vi "HW_GEN - Read DevicesInfo from XML File.vi"(8 "error in":errorcluster caption="错误输入（无错误）", 11 "path to XML document":path=path "E:/00. 系统集成/000000 SignalPro/SourceCodes/Builds/Files/HWdef.xml" caption="XML文档路径") -> (0 "error out":errorcluster caption="错误输出", 2 "DevInfo[]":T1[](array[typedef]))   [LabVIEW 2016]
uses:
  <vilib>/xml/NI_XML.lvlib
  Ctrls/HardWare Basic Info _ Channel.ctl
  Ctrls/HardWare Basic Info _ Module.ctl
  Ctrls/HardWare Basic Info _ Chassis.ctl
  Ctrls/HardWare Basic Info _ Device.ctl
  <vilib>/xml/Load XML File.vi
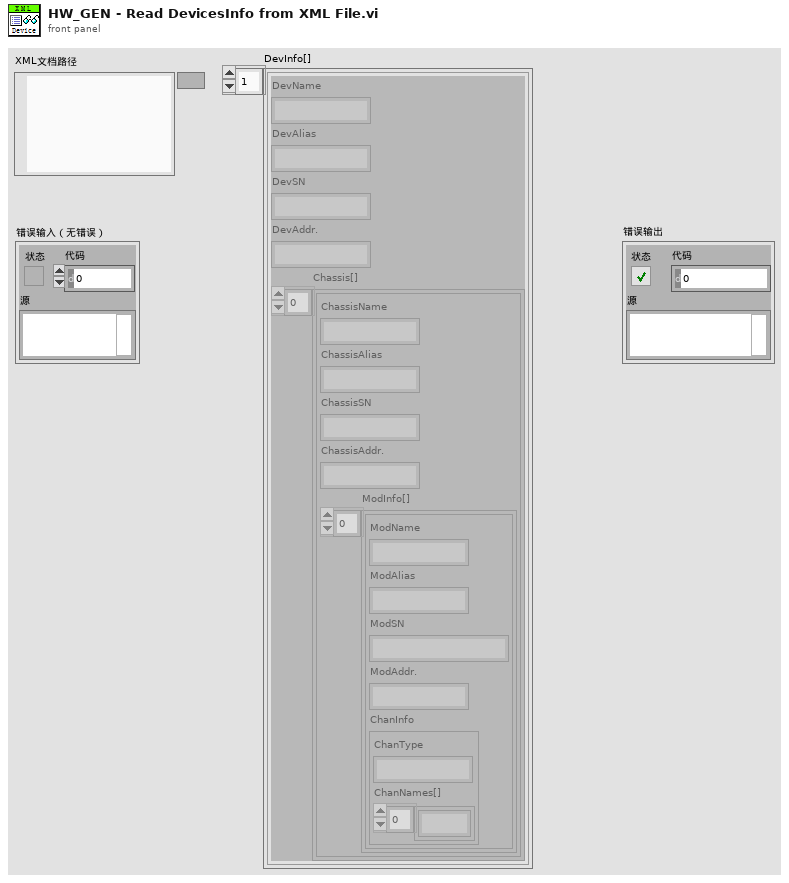
[diagram p1: front panel]
types:
  T1 = typedef "HardWare Basic Info _ Device.ctl" = cluster{"DevName":string, "DevAlias":string, "DevSN":string, "DevAddr.":string, "Chassis[]":T2[]}
  T2 = typedef "HardWare Basic Info _ Chassis.ctl" = cluster{"ChassisName":string, "ChassisAlias":string, "ChassisSN":string, "ChassisAddr.":string, "ModInfo[]":T3[]}
  T3 = typedef "HardWare Basic Info _ Module.ctl" = cluster{"ModName":string, "ModAlias":string, "ModSN":string, "ModAddr.":string, "ChanInfo":T4}
  T4 = typedef "HardWare Basic Info _ Channel.ctl" = cluster{"ChanType":string, "ChanNames[]":string[]}
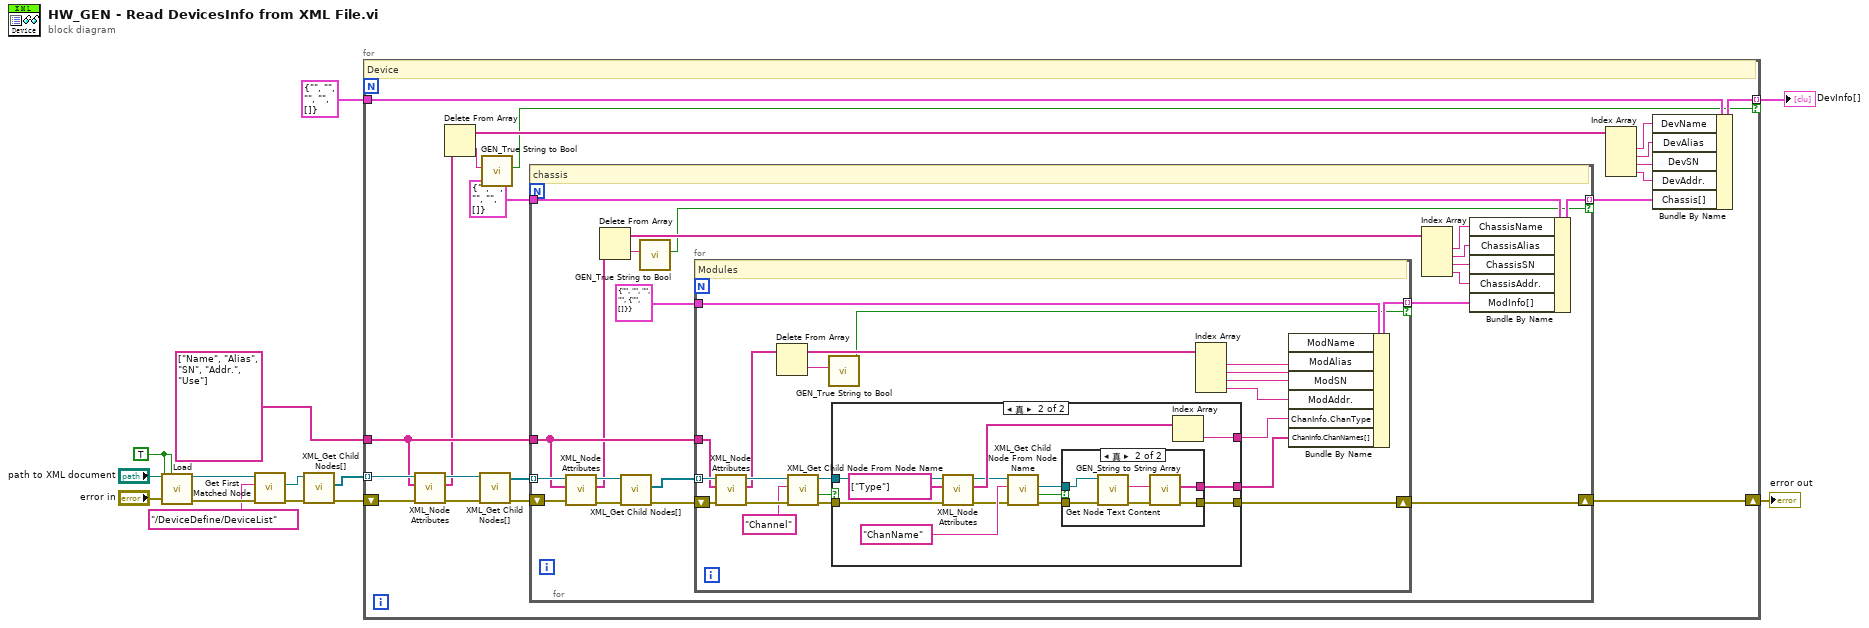
[diagram p0: block diagram]
diagram:
  w1 = TRUE ("process namespaces (False)")
  n1 = call-poly <vilib>:"Load.vi"("path to XML document"="path to XML document", "preserve whitespace (True)"=w1, "process namespaces (False)"=w1, "error in (no error)"="error in") -> ("DOM document out"=w11:refnum<k20>, "error out"=w13:errorcluster)  [unwired: 9 in, 1 out]
  n2 = call <vilib>:"Get First Matched Node.vi"("error in (no error)"=w13, "XPath expression"="/DeviceDefine/DeviceList", "node in"=w11) -> ("error out"=w9:errorcluster, "node result"=w10:refnum<k20>)  [unwired: 6 in, 1 out]
  n3 = call "XML_Get Child Nodes[].vi"("错误输入（无错误）"=w9, "ref in"=w10) -> ("错误输出"=w7:errorcluster, "ElementChildNod[]"=w8:refnum<k20>[])  [unwired: 6 in, 2 out]
  n4 = for {
    tunnel: w8 -> [w34] mode=indexing
    shift-right: [w30] -> w4
    shift-left: w7 -> [w33]
    tunnel: T1 {"DevName"="", "DevAlias"="", "DevSN"="", "DevAddr."="", "Chassis[]"=[]} ("Device") -> [w32]
    tunnel: [w29] -> w5 mode=indexing if=w16
    tunnel: string[] ["Name", "Alias", "SN", "Addr.", "Use"] ("AttributeNames") -> [w27]
    # "Device"
    n5 = call "XML_Node Attributes.vi"("error in"=w33, "AttributeNames"=w27, "node in"=w34) -> ("error out"=w31:errorcluster, "Values"=w26:string[], "node out"=w28:refnum<k20>)  [unwired: 6 in]
    n6 = Delete From Array(array=w26) -> (deleted portion=w24:string, array with subset deleted=w25:string[])  [unwired: 2 in]
    n7 = call "XML_Get Child Nodes[].vi"("错误输入（无错误）"=w31, "ref in"=w28) -> ("错误输出"=w19:errorcluster, "ElementChildNod[]"=w20:refnum<k20>[])  [unwired: 6 in, 2 out]
    n8 = call "GEN_True String to Bool.vi"("string in"=w24) -> ("true?"=w16:bool)  [unwired: 10 in]
    n9 = for {
      tunnel: w20 -> [w53] mode=indexing
      tunnel: T2 {"ChassisName"="", "ChassisAlias"="", "ChassisSN"="", "ChassisAddr."="", "ModInfo[]"=[]} ("Chassis") -> [w49]
      shift-right: [w43] -> w30
      shift-left: w19 -> [w54]
      tunnel: [w42] -> w17 mode=indexing if=w36
      tunnel: w27 -> [w40]
      # "chassis"
      n10 = call "XML_Node Attributes.vi"("error in"=w54, "AttributeNames"=w40, "node in"=w53) -> ("error out"=w48:errorcluster, "Values"=w39:string[], "node out"=w41:refnum<k20>)  [unwired: 6 in]
      n11 = Delete From Array(array=w39) -> (deleted portion=w37:string, array with subset deleted=w38:string[])  [unwired: 2 in]
      n12 = call "XML_Get Child Nodes[].vi"("错误输入（无错误）"=w48, "ref in"=w41) -> ("错误输出"=w47:errorcluster, "ElementChildNod[]"=w46:refnum<k20>[])  [unwired: 6 in, 2 out]
      n13 = call "GEN_True String to Bool.vi"("string in"=w37) -> ("true?"=w36:bool)  [unwired: 10 in]
      n14 = for {
        shift-right: [w66] -> w43
        shift-left: w47 -> [w75]
        tunnel: w46 -> [w76] mode=indexing
        tunnel: T3 {"ModName"="", "ModAlias"="", "ModSN"="", "ModAddr."="", "ChanInfo"={"ChanType"="", "ChanNames[]"=[]}} ("ModInfo") -> [w71]
        tunnel: [w70] -> w44 mode=indexing if=w56
        tunnel: w40 -> [w64]
        # "Modules"
        n15 = call "XML_Node Attributes.vi"("error in"=w75, "AttributeNames"=w64, "node in"=w76) -> ("error out"=w69:errorcluster, "Values"=w59:string[], "node out"=w65:refnum<k20>)  [unwired: 6 in]
        n16 = Delete From Array(array=w59) -> (deleted portion=w57:string, array with subset deleted=w58:string[])  [unwired: 2 in]
        n17 = call "XML_Get Child Node From Node Name.vi"("error in"=w69, "NodeName"="Channel" ("名称"), "ref in"=w65) -> ("错误输出"=w68:errorcluster, "find?"=w60:bool, "subNode out"=w67:refnum<k20>)  [unwired: 6 in]
        n18 = call "GEN_True String to Bool.vi"("string in"=w57) -> ("true?"=w56:bool)  [unwired: 10 in]
        n19 = case shown="真" w60 {
          tunnel: w68 -> [w77 w90]
          tunnel: w67 -> [_ w89]
          tunnel: [w77 w88] -> w66
          tunnel: [_ w79] -> w62
          tunnel: [_ w78] -> w61
          frame False {
          }
          frame True {
            n20 = call "XML_Node Attributes.vi"("error in"=w90, "AttributeNames"=string[] ["Type"], "node in"=w89) -> ("error out"=w83:errorcluster, "Values"=w85:string[], "node out"=w84:refnum<k20>)  [unwired: 6 in]
            n21 = call "XML_Get Child Node From Node Name.vi"("error in"=w83, "NodeName"="ChanName" ("名称"), "ref in"=w84) -> ("错误输出"=w81:errorcluster, "find?"=w82:bool, "subNode out"=w80:refnum<k20>)  [unwired: 6 in]
            n22 = case shown="真" w82 {
              tunnel: w81 -> [w91 w94]
              tunnel: w80 -> [_ w96]
              tunnel: [w91 w93] -> w88
              tunnel: [_ w95] -> w78
              frame False {
              }
              frame True {
                n23 = call <vilib>:"Get Node Text Content.vi"("error in (no error)"=w94, "node in"=w96) -> ("error out"=w93:errorcluster, "node text"=w92:string)  [unwired: 7 in, 1 out]
                n24 = call "GEN_String to String Array.vi"("String in"=w92) -> ("String Array out"=w95:string[])  [unwired: 10 in]
              }
            }
            n25 = Index Array(array=w85) -> (element=w79:string)  [unwired: 1 in]
          }
        }
        n26 = Index Array(array=w58) -> (element #1=w72:string, element #2=w73:string, element #3=w74:string, element #4=w55:string)  [unwired: 4 in]
        n27 = Bundle By Name(cluster=w71, "ModName"=w72, "ModAlias"=w73, "ModSN"=w74, "ModAddr."=w55, "ChanInfo.ChanType"=w62, "ChanInfo.ChanNames[]"=w61) -> (w70:T3)
      }
      n28 = Index Array(array=w38) -> (element #1=w52:string, element #2=w51:string, element #3=w50:string, element #4=w35:string)  [unwired: 4 in]
      n29 = Bundle By Name(cluster=w49, "ChassisName"=w52, "ChassisAlias"=w51, "ChassisSN"=w50, "ChassisAddr."=w35, "ModInfo[]"=w44) -> (w42:T2)
    }
    n30 = Index Array(array=w25) -> (element #1=w21:string, element #2=w22:string, element #3=w23:string, element #4=w15:string)  [unwired: 4 in]
    n31 = Bundle By Name(cluster=w32, "DevName"=w21, "DevAlias"=w22, "DevSN"=w23, "DevAddr."=w15, "Chassis[]"=w17) -> (w29:T1)
  }
  "DevInfo[]" <- w5
  "error out" <- w4
